vi "Read.vi"(7 "I2C Channel (0)":u8, 8 "Error In":errorcluster, 9 "Resolution":enum16{"2g", "4g", "8g", "16g"}(ring), 10 "I2C Slave Address":T2, 11 "LINX Resource":T3) -> (0 "Error Out":errorcluster, 2 "Acceleration Data (g)":T1, 3 "LINX Resource":T3)   [LabVIEW 2020, in "LMH-LINX.lvlib" / "ADXL345.lvlib"]
doc: "Read X, Y and Z axis of acceleration data (in g's) from the ADXL345."
uses:
  ADXL345.lvlib
  Private/Type Defs/LINX Ref.ctl
  Private/Type Defs/Platform.ctl
  Private/Type Defs/Interface.ctl
  Private/Device/Type Defs/LINX Device Config.ctl
  Private/Device/Type Defs/TCP Config.ctl
  Private/Device/Type Defs/Channels.ctl
  Address.ctl
  Private/Local IO/LinxI2cWrite.vi
  Utilities/Check Channel.vi
  Private/Utilties/Generate Error.vi
  LMH-LINX.lvlib
  Toolbox/LMH-Toolbox.lvlib
  Private/Device/Device.lvlib
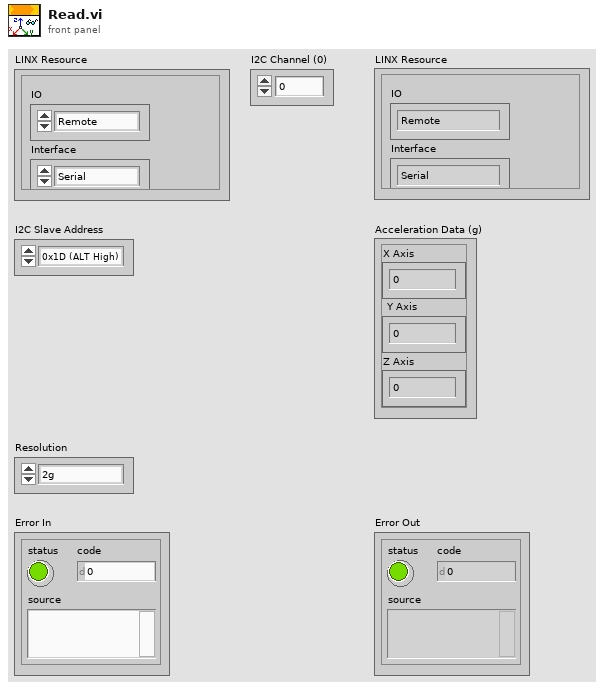
[diagram p1: front panel]
types:
  T1 = cluster{"X Axis":dbl, "Y Axis":dbl, "Z Axis":dbl}
  T2 = typedef "LMH-LINX.lvlib/ADXL345.lvlib/Address.ctl" = enum16{"0x1D (ALT High)", "0x53 (ALT Low)"}
  T3 = typedef "LMH-LINX.lvlib/LINX Ref.ctl" = cluster{"IO":T4, "Interface":T5, "LINX Device Config":T6}
  T4 = typedef "LMH-LINX.lvlib/Platform.ctl" = enum16{"Remote", "Local"}
  T5 = typedef "LMH-LINX.lvlib/Interface.ctl" = enum16{"Serial", "TCP"}
  T6 = typedef "LMH-LINX.lvlib/Device.lvlib/LINX Device Config.ctl" = cluster{"Interface":T5, "COM Port":refnum<visa-resource-name>, "TCP Configuration":T7, "Device Family":u8, "Device ID":u8, "Device Name":string, "TCP Ref":refnum<k5>, "Channels":T8}
  T7 = typedef "LMH-LINX.lvlib/Device.lvlib/TCP Config.ctl" = cluster{"IP Address":string, "Port":u16}
  T8 = typedef "LMH-LINX.lvlib/Channels.ctl" = cluster{"DI":u8[], "DO":u8[], "AI":u8[], "AO":u8[], "PWM":u8[], "QE":u8[], "UART":u8[], "I2C 2":u8[], "SPI":u8[], "CAN":u8[], "Servo":u8[], "AI Ref (V)":dbl, "AI Resolution (Bits)":u8, "AO Ref (V)":dbl, "AO Resolution (Bits)":u8}
  T9 = cluster{"Decimal I16":i16, "Decimal I16":i16, "Decimal I16":i16}
  T10 = cluster{"Decimal I16":dbl, "Decimal I16":dbl, "Decimal I16":dbl}
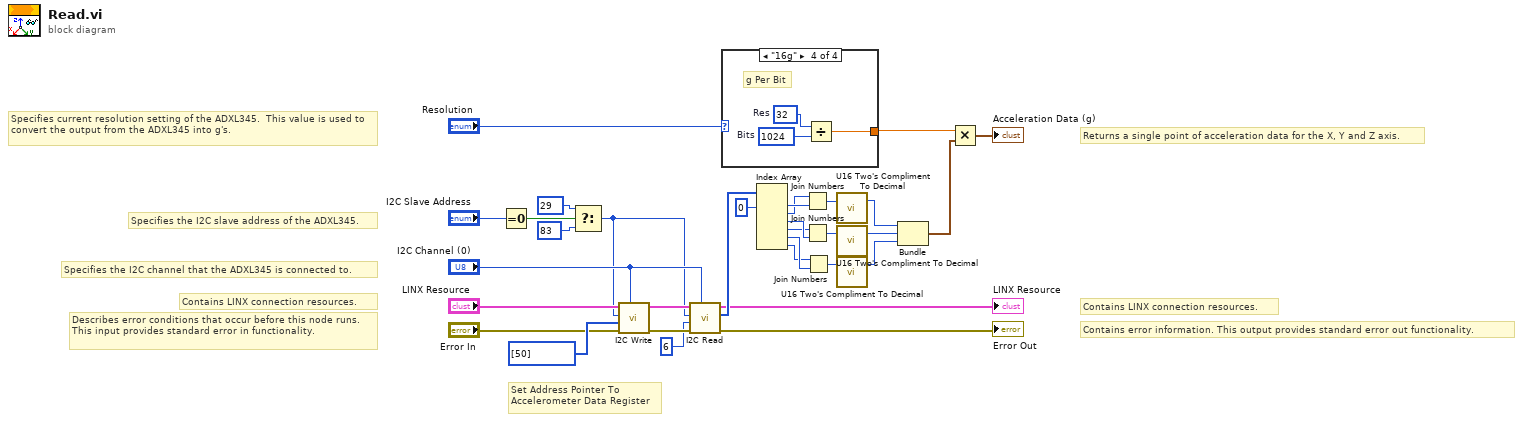
[diagram p0: block diagram]
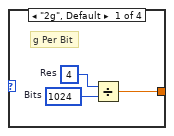
[diagram p2: hidden frame]
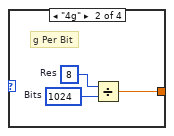
[diagram p3: hidden frame]
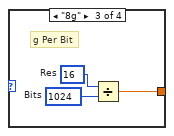
[diagram p4: hidden frame]
diagram:
  # "Returns a single point of acceleration data for the X, Y and Z axis."
  # "Contains LINX connection resources."
  # "Contains error information. This output provides standard error out functionality."
  # "Specifies current resolution setting of the ADXL345.  This value is used to convert the output from the ADXL345 into g's."
  # "Specifies the I2C slave address of the ADXL345."
  # "Specifies the I2C channel that the ADXL345 is connected to."
  # "Contains LINX connection resources."
  # "Describes error conditions that occur before this node runs. This input provides standard error in functionality."
  # "Set Address Pointer To \nAccelerometer Data Register"
  n1 = Equal To 0?(x="I2C Slave Address") -> (x = 0?=w32:bool)
  n2 = Select(t=u8 29 ("I2C Slave Address (0)"), s=w32, f=u8 83 ("I2C Slave Address (0)")) -> (s? t:f=w22:u8)
  n3 = call "I2C Write.vi"("I2C Channel"="I2C Channel (0)", "Error In"="Error In", "Data"=u8[] [50], "I2C Slave Address (0)"=w22, "LINX Resource"="LINX Resource") -> ("Error Out"=w24:errorcluster, "LINX Resource"=w25:T3)  [unwired: 5 in]
  n4 = call "I2C Read.vi"("I2C Channel"="I2C Channel (0)", "Error In"=w24, "Bytes To Read"=u8 6, "I2C Slave Address (0)"=w22, "LINX Resource"=w25) -> ("Error Out"=→"Error Out":errorcluster, "Data"=w20:u8[], "LINX Resource"=→"LINX Resource":T3)  [unwired: 4 in]
  n5 = case shown="\"16g\"" "Resolution" {
    tunnel: [w33 w36 w39 w42] -> w4
    frame "2g", Default {
      w34 = 4  # Res
      w35 = 1024  # Bits
      # "g Per Bit"
      n6 = Divide(x=w34, y=w35) -> (x/y=w33:dbl)
    }
    frame "4g" {
      w37 = 8  # Res
      w38 = 1024  # Bits
      # "g Per Bit"
      n7 = Divide(x=w37, y=w38) -> (x/y=w36:dbl)
    }
    frame "8g" {
      w40 = 16  # Res
      w41 = 1024  # Bits
      # "g Per Bit"
      n8 = Divide(x=w40, y=w41) -> (x/y=w39:dbl)
    }
    frame "16g" {
      w43 = 32  # Res
      w44 = 1024  # Bits
      # "g Per Bit"
      n9 = Divide(x=w43, y=w44) -> (x/y=w42:dbl)
    }
  }
  n10 = Index Array(array=w20, index #1=0 ("index")) -> (element #1=w16:u8, element #2=w15:u8, element #3=w14:u8, element #4=w13:u8, element #5=w12:u8, element #6=w11:u8)  [unwired: 5 in]
  n11 = Join Numbers(hi=w15, lo=w16) -> ((hi.lo)=w10:u16)
  n12 = Join Numbers(hi=w13, lo=w14) -> ((hi.lo)=w9:u16)
  n13 = Join Numbers(hi=w11, lo=w12) -> ((hi.lo)=w8:u16)
  n14 = call "U16 Two's Compliment To Decimal.vi"("Two's Compliment U16"=w10) -> ("Decimal I16"=w7:i16)  [unwired: 2 in]
  n15 = call "U16 Two's Compliment To Decimal.vi"("Two's Compliment U16"=w9) -> ("Decimal I16"=w6:i16)  [unwired: 2 in]
  n16 = call "U16 Two's Compliment To Decimal.vi"("Two's Compliment U16"=w8) -> ("Decimal I16"=w5:i16)  [unwired: 2 in]
  n17 = Bundle("Decimal I16"=w7, "Decimal I16"=w6, "Decimal I16"=w5) -> (w3:T9)  [unwired: 1 in]
  n18 = Multiply(x=w4, y=w3) -> (x*y=→"Acceleration Data (g)":T10)
